vi "Execute.vi"(8 "error in (no error)":errorcluster, 9 "M1M3 Support Events in":refnum<class "M1M3 Support Events.lvclass">, 11 "Controller in":refnum<class "Controller.lvclass">) -> (0 "error out":errorcluster, 3 "Controller out":refnum<class "Controller.lvclass">)   [LabVIEW 2016, in "Controller.lvclass"]
uses:
  Controller.lvclass
  M1M3 Support Events/M1M3 Support Events.lvclass
  M1M3 Support Events/M1M3 Support Events.lvclass/M1M3 Support Events.ctl
  Typedefs/StateTypes.ctl
  SAL/SAL.lvclass
  Typedefs/M1M3SupportEUI_TypeDefs.lvlib
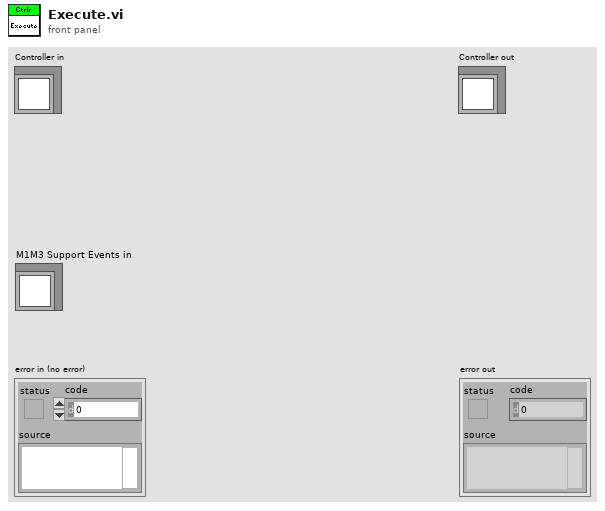
[diagram p1: front panel]
types:
  T1 = typedef "M1M3SupportEUI_TypeDefs.lvlib/M1M3 Support Events.ctl" = cluster{"M1M3 Support State":refnum<user-event>, "Inclinometer  Data":refnum<user-event>, "IMS Data":refnum<user-event>}
  T2 = typedef "M1M3SupportEUI_TypeDefs.lvlib/StateTypes.ctl" = enum16{"Offline State", "Fault State", "Standby State", "Disabled State", "Enabled State", "Wait For User Input State", "Test Actuator State"}
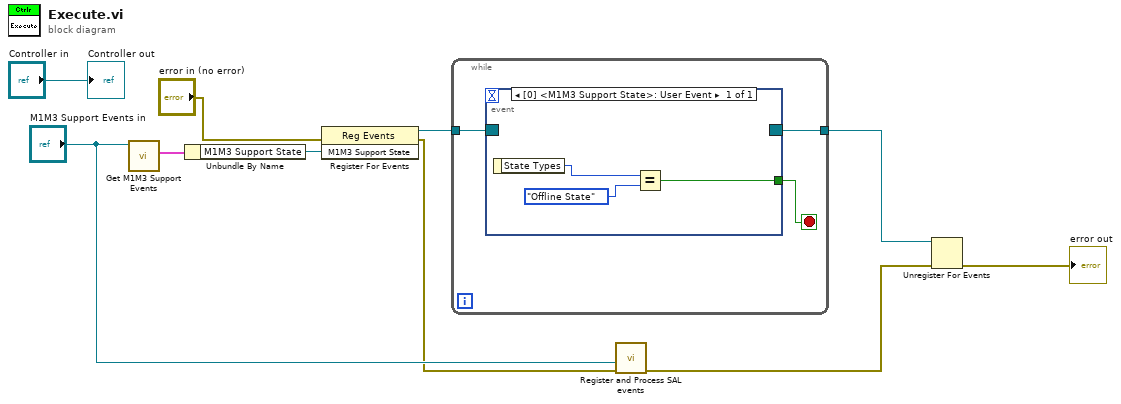
[diagram p0: block diagram]
diagram:
  n1 = call "Get M1M3 Support Events.vi"("M1M3 Support Events in"="M1M3 Support Events in") -> ("M1M3 Support Events"=w7:T1)  [unwired: 9 in, 1 out]
  n2 = Unbundle By Name(w7) -> ("M1M3 Support State"=w6:refnum<user-event>)
  n3 = register-events(error in="error in (no error)", w6) -> (reference out=w3:refnum<event-registration>, error out=w4:errorcluster)  [unwired: 1 in]
  n4 = while {
    tunnel: w3 -> [w13]
    tunnel: [w12] -> w2
    stop <- w11 stop-if-true
    n5 = event shown="[0] <M1M3 Support State>: User Event" {
      selector: w13 -> [_]
      dyn-events: [_] -> w12
      timeout: _ -> [_]
      tunnel: [w14] -> w11
      event User Event {
        n6 = event-data() -> ("State Types"=w16:T2)  [unwired: 1 in]
        n7 = Equal?(x=w16, y=StateTypes."Offline State" ("State Types")) -> (x = y?=w14:bool)
      }
    }
  }
  n8 = call "Register and Process SAL events.vi"("error in (no error)"=w4, "M1M3 Support Events in"="M1M3 Support Events in") -> ("error out"=w1:errorcluster)  [unwired: 8 in, 1 out]
  n9 = Unregister For Events(event registration refnum=w2, error in=w1) -> (error out=→"error out":errorcluster)
  "Controller out" <- "Controller in"
